vi "Generate Async Cmd Event.vi"(7 "AdHoc Cmd (\"\")":string, 8 "error in (no error)":errorcluster, 9 "vData":variant, 10 "AsyncCmd":T1, 11 "DLP2 in":refnum<class "DLP2.lvclass">) -> (0 "error out":errorcluster, 3 "DLP2 out":refnum<class "DLP2.lvclass">)   [LabVIEW 2022 SP3, in "DLP2.lvclass"]
doc: "Developed by Kevin Thompson\nkevin@thompsonengineering.net\n\nCopyright 2018\nThompson Engineering, LLC"
uses:
  DLP2.lvclass
  DLP2.lvclass/DLP2.ctl
  Common/Controls/TD Async CmdMsg EventData--cluster.ctl
  DataTypes/AsynCmd_Temp01--enum.ctl
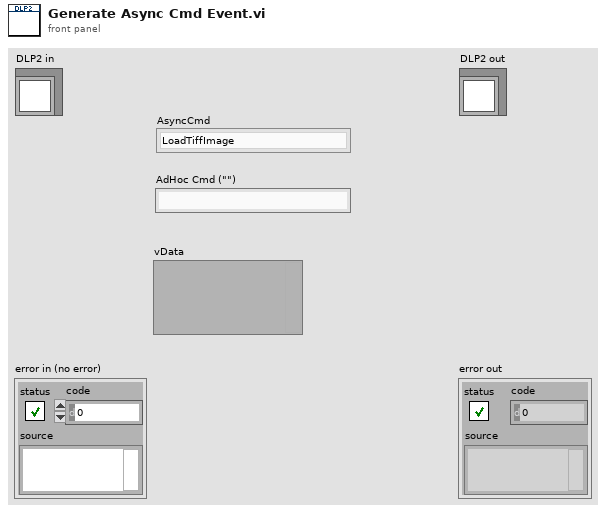
[diagram p1: front panel]
types:
  T1 = typedef "DLP2.lvclass/AsynCmd_Temp01--enum.ctl" = enum16{"LoadTiffImage"}
  T2 = typedef "TD Async CmdMsg EventData--cluster.ctl" = cluster{"Time Stamp":timestamp, "CmdMsg":string, "vData":variant}
  T3 = typedef "DLP2.lvclass/Public Events--cluster.ctl" = cluster{"Temp01.AsyncCmd Event":refnum<user-event>, "Temp01.AsyncMsg Event":refnum<user-event>, "stop process":refnum<user-event>, "API Incoming Event":refnum<user-event>, "API Executed Event":refnum<user-event>, "API Return Event":refnum<user-event>}
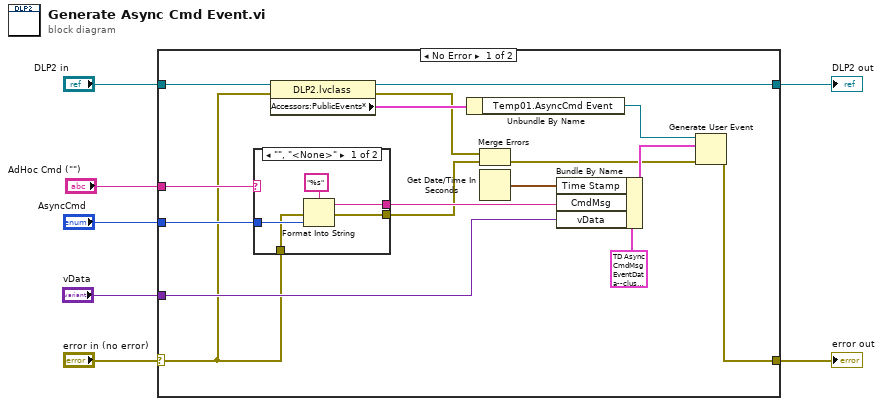
[diagram p0: block diagram]
diagram:
  n1 = case shown="No Error" "error in (no error)" {
    selector: "error in (no error)" -> [w10 w32]
    tunnel: [w23 w32] -> w6
    tunnel: [w13 w31] -> w4
    tunnel: "DLP2 in" -> [w17 w31]
    tunnel: "AsyncCmd" -> [w15 _]
    tunnel: "vData" -> [w18 _]
    tunnel: "AdHoc Cmd (\"\")" -> [w14 _]
    frame No Error {
      n2 = case shown="\"\", \"<None>\"" w14 {
        selector: w14 -> [_ w29]
        tunnel: w15 -> [w27 _]
        tunnel: [w26 w29] -> w19
        tunnel: w10 -> [w25 w30]
        tunnel: [w24 w30] -> w16
        frame "", "<None>" {
          n3 = Format Into String(format string="%s", error in=w25, w27) -> (resulting string=w26:string, error out=w24:errorcluster)  [unwired: 1 in]
        }
        frame Default {
        }
      }
      n4 = property class="DLP2.lvclass"(reference=w17, error in=w10) -> (reference out=w13:refnum<class "DLP2.lvclass">, error out=w8:errorcluster, "Accessors:PublicEvents*"=w12:T3)
      n5 = Unbundle By Name(w12) -> ("Temp01.AsyncCmd Event"=w11:refnum<user-event>)
      n6 = Merge Errors(w8, w16) -> (w9:errorcluster)
      n7 = Get Date/Time In Seconds() -> (seconds since 1Jan1904=w20:timestamp)
      n8 = Bundle By Name(cluster=T2 {"Time Stamp"=timestamp(0 s since 1904-01-01), "CmdMsg"="", "vData"=variant} ("Async EvData"), "Time Stamp"=w20, "CmdMsg"=w19, "vData"=w18) -> (w22:T2)
      n9 = Generate User Event(user event=w11, event data cluster=w22, error in=w9) -> (error out=w23:errorcluster)  [unwired: 1 in, 1 out]
    }
    frame Error {
    }
  }
  "error out" <- w6
  "DLP2 out" <- w4
